vi "SineWave.vi"(8 "error in (no error)":errorcluster, 9 "DC Offset":dbl, 10 "Amplitude":dbl, 11 "Amount of points":i32) -> (0 "error out":errorcluster, 3 "Array":dbl[](array[numeric]))   [LabVIEW 2020]
panel:
  out "Waveform Graph":dbl[](graph)
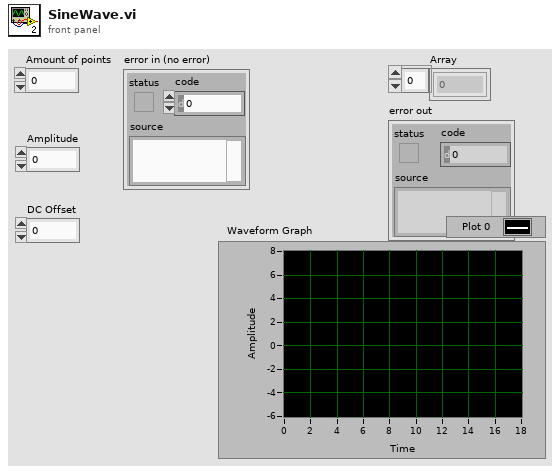
[diagram p1: front panel]
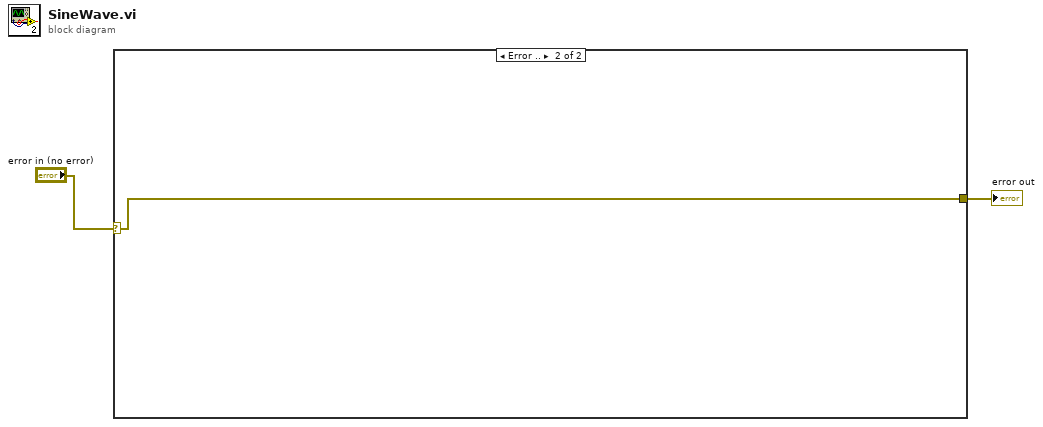
[diagram p0: block diagram]
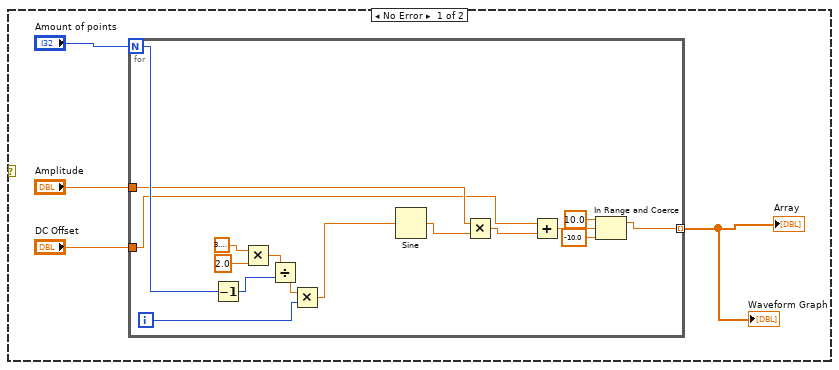
[diagram p2: hidden frame]
diagram:
  n1 = case shown="Error .." "error in (no error)" {
    selector: "error in (no error)" -> [_ w23]
    tunnel: [_ w23] -> w1
    frame No Error {
      n2 = for {
        N: "Amount of points" -> [w16]
        tunnel: "Amplitude" -> [w13]
        tunnel: "DC Offset" -> [w11]
        tunnel: [w7] -> w3 mode=indexing
        i -> [w21]
        n3 = Decrement(x=w16) -> (x-1=w15:i32)
        n4 = Multiply(x=3.141592653589793, y=2.0) -> (x*y=w19:dbl)
        n5 = Divide(x=w19, y=w15) -> (x/y=w18:dbl)
        n6 = Multiply(x=w18, y=w21) -> (x*y=w20:dbl)
        n7 = Sine(x=w20) -> (sin(x)=w14:dbl)
        n8 = Multiply(x=w13, y=w14) -> (x*y=w12:dbl)
        n9 = Add(x=w11, y=w12) -> (x+y=w10:dbl)
        n10 = In Range and Coerce(upper limit=10.0, x=w10, lower limit=-10.0) -> (coerced(x)=w7:dbl)  [unwired: 1 out]
      }
      "Array" <- w3
      "Waveform Graph" <- w3
    }
    frame Error {
    }
  }
  "error out" <- w1
